vi "Flatten Value.vi"(8 "error in (no error)":errorcluster, 11 "Boolean in":refnum<class "Assertion 1D.lvclass">) -> (0 "error out":errorcluster, 2 "Value":string, 3 "Boolean out":refnum<class "Assertion 1D.lvclass">)   [LabVIEW 2020, in "Assertion 1D.lvclass"]
uses:
  <vilib>/gpm_packages/@cs/data-type-serializer/source/Assertion 1D/Assertion 1D.lvclass
  <vilib>/gpm_packages/@cs/data-type-serializer/source/Assertion 1D/Assertion 1D.lvclass/Assertion 1D.ctl
  <vilib>/gpm_packages/@cs/run-time-assertions/Source/Assert/Assert.lvclass
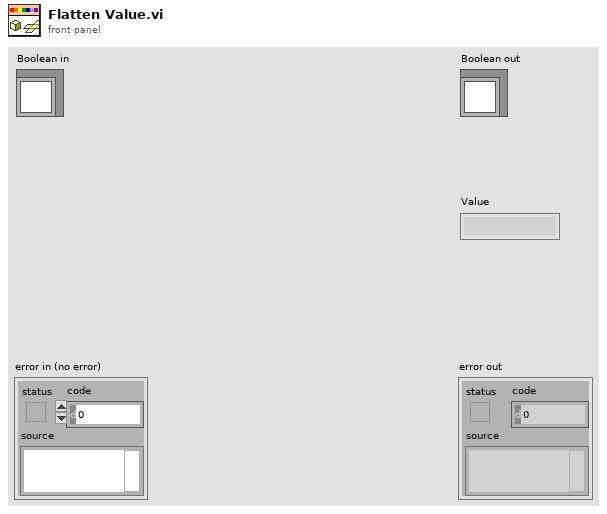
[diagram p1: front panel]
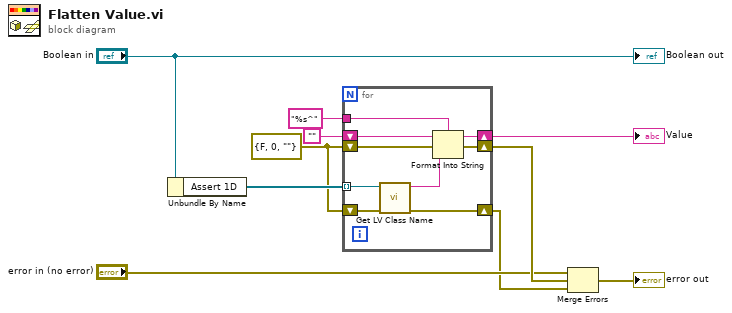
[diagram p0: block diagram]
diagram:
  w2 = errorcluster {"status"=FALSE, "code"=0, "source"=""} ("error IO")
  n1 = Unbundle By Name("Boolean in") -> ("Assert 1D"=w9:refnum<class "Assert.lvclass">[])
  n2 = for {
    tunnel: w9 -> [w14] mode=indexing
    shift-right: [w19] -> w8
    shift-left: "" -> [w17]
    tunnel: "%s^" ("delimiter (Tab)") -> [w16]
    shift-right: [w18] -> w7
    shift-left: w2 -> [w15]
    shift-right: [w11] -> w1
    shift-left: w2 -> [w12]
    n3 = call <vilib>:"Get LV Class Name.vi"("error in (no error)"=w12, "object"=w14) -> ("error out"=w11:errorcluster, "class name"=w13:string)  [unwired: 8 in]
    n4 = Format Into String(format string=w16, initial string=w17, error in=w15, w13) -> (resulting string=w19:string, error out=w18:errorcluster)
  }
  "Value" <- w8
  n5 = Merge Errors("error in (no error)", w7, w1) -> (→"error out":errorcluster)
  "Boolean out" <- "Boolean in"
